vi "ComputePoint.vi"(7 "Calibration":T2={"XHP ChirpGain"=1.0, "YHP ChirpGain"=1.0, "XLP ChirpGain"=1.0, "YLP ChirpGain"=1.0}, 8 "LP Center Frequency":u32=805306367 format="%x", 9 "HP Center Frequency":u32=805306367 format="%x", 10 "UpdatesPerPoint":u32, 11 "Point":cluster{"X":i32, "Y":i32, "Z":i32} {"Y" format="%x"; "X" format="%x"}) -> (3 "settings":T1)   [LabVIEW 2011]
uses:
  AODCalibration.ctl
  CoordinateSettings.ctl
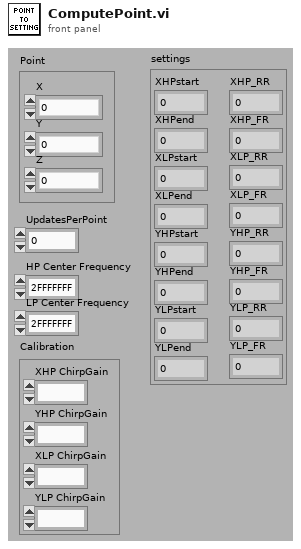
[diagram p1: front panel]
types:
  T1 = typedef "CoordinateSettings.ctl" = cluster{"XHPstart":u32, "XHPend":u32, "XLPstart":u32, "XLPend":u32, "YHPstart":u32, "YHPend":u32, "YLPstart":u32, "YLPend":u32, "XHP_RR":u32, "XHP_FR":u32, "XLP_FR":u32, "XLP_RR":u32, "YHP_FR":u32, "YHP_RR":u32, "YLP_FR":u32, "YLP_RR":u32}
  T2 = typedef "AODCalibration.ctl" = cluster{"XHP ChirpGain":fxp<+/-,16,2>, "YHP ChirpGain":fxp<+/-,16,2>, "XLP ChirpGain":fxp<+/-,16,2>, "YLP ChirpGain":fxp<+/-,16,2>}
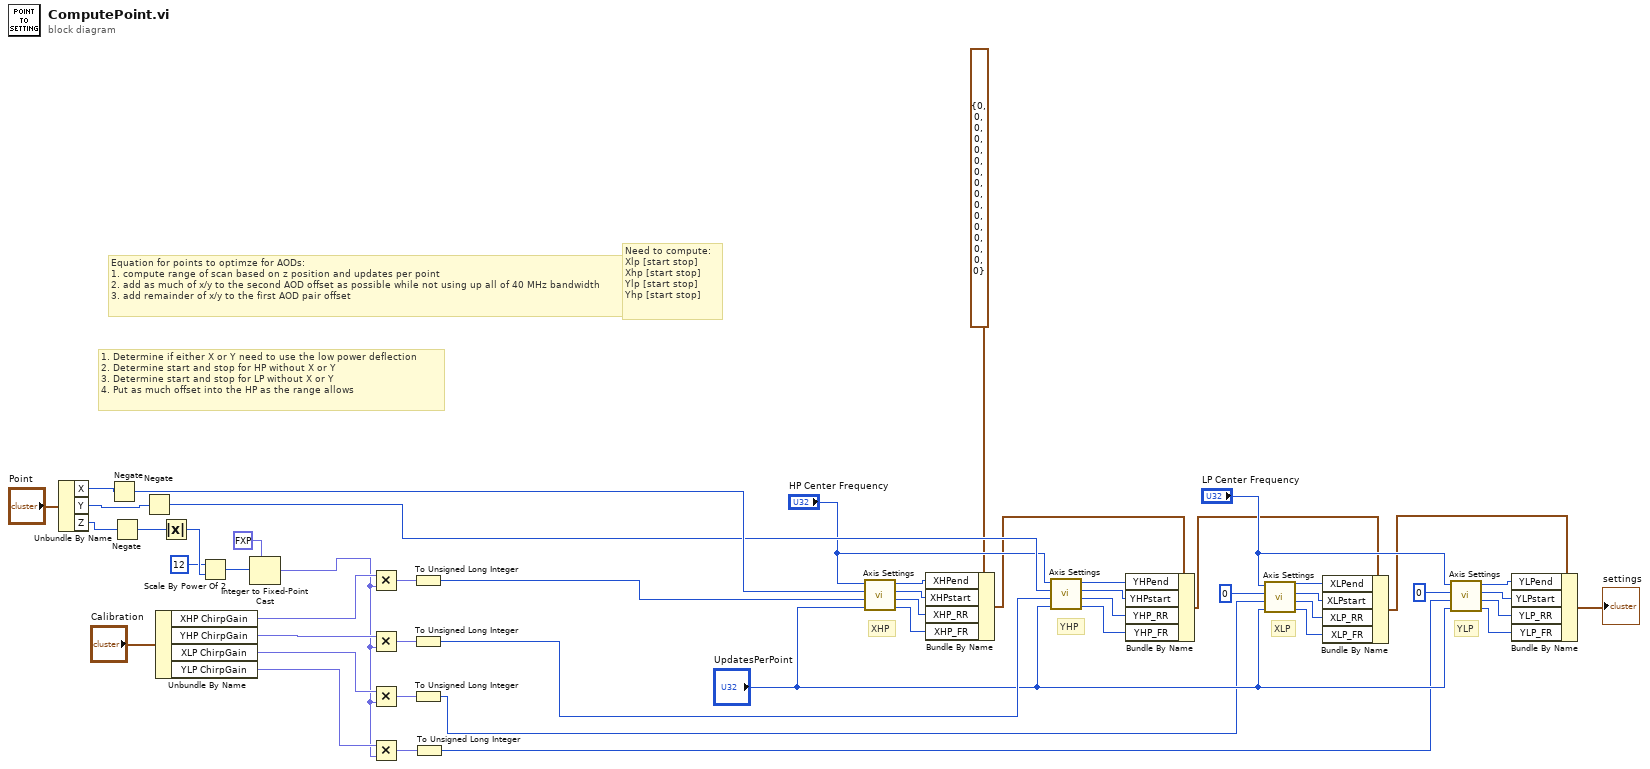
[diagram p0: block diagram]
diagram:
  # "YLP"
  # "XLP"
  # "YHP"
  # "XHP"
  # "1. Determine if either X or Y need to use the low power deflection\n2. Determine start and stop for HP without X or Y\n3. Determine start and stop for LP without X or Y\n4. Put as much offset into the HP as the range allows"
  # "Need to compute:\nXlp [start stop]\nXhp [start stop]\nYlp [start stop]\nYhp [start stop]"
  # "Equation for points to optimze for AODs:\n1. compute range of scan based on z position and updates per point\n2. add as much of x/y to the second AOD offset as possible while not using up all of 40 MHz bandwidth\n3. add remainder of x/y to the first AOD pair offset"
  n1 = Unbundle By Name("Point") -> ("X"=w50:i32, "Y"=w49:i32, "Z"=w48:i32)
  n2 = Negate(x=w50) -> (-x=w37:i32)
  n3 = Negate(x=w48) -> (-x=w42:i32)
  n4 = Negate(x=w49) -> (-x=w36:i32)
  n5 = Unbundle By Name("Calibration") -> ("XHP ChirpGain"=w46:fxp<+/-,16,2>, "YHP ChirpGain"=w45:fxp<+/-,16,2>, "XLP ChirpGain"=w44:fxp<+/-,16,2>, "YLP ChirpGain"=w43:fxp<+/-,16,2>)
  n6 = Absolute Value(x=w42) -> (abs(x)=w5:i32)
  n7 = Scale By Power Of 2(n=12, x=w5) -> (x*2^n=w3:i32)
  n8 = Integer to Fixed-Point Cast(fixed-point type=fxp<+/-,32,20> 0.0, integer=w3) -> (fixed-point=w2:fxp<+/-,32,20>)
  n9 = Multiply(x=w46, y=w2) -> (x*y=w41:fxp<+/-,48,22>)
  n10 = Multiply(x=w45, y=w2) -> (x*y=w40:fxp<+/-,48,22>)
  n11 = Multiply(x=w44, y=w2) -> (x*y=w39:fxp<+/-,48,22>)
  n12 = Multiply(x=w43, y=w2) -> (x*y=w38:fxp<+/-,48,22>)
  n13 = To Unsigned Long Integer(number=w41) -> (unsigned 32bit integer=w29:u32)
  n14 = To Unsigned Long Integer(number=w40) -> (unsigned 32bit integer=w28:u32)
  n15 = To Unsigned Long Integer(number=w39) -> (unsigned 32bit integer=w24:u32)
  n16 = To Unsigned Long Integer(number=w38) -> (unsigned 32bit integer=w22:u32)
  n17 = call "Axis Settings.vi"("Updates Per Point"="UpdatesPerPoint", "Ramp"=w29, "Offset"=w37, "Center Frequency"="HP Center Frequency") -> ("Falling Rate"=w30:u32, "Rising Rate"=w31:u32, "Low"=w32:u32, "High"=w33:u32)  [unwired: 4 in]
  n18 = Bundle By Name(cluster=T1 {"XHPstart"=0, "XHPend"=0, "XLPstart"=0, "XLPend"=0, "YHPstart"=0, "YHPend"=0, "YLPstart"=0, "YLPend"=0, "XHP_RR"=0, "XHP_FR"=0, "XLP_FR"=0, "XLP_RR"=0, "YHP_FR"=0, "YHP_RR"=0, "YLP_FR"=0, "YLP_RR"=0} ("settings"), "XHPend"=w33, "XHPstart"=w32, "XHP_RR"=w31, "XHP_FR"=w30) -> (w17:T1)
  n19 = call "Axis Settings.vi"("Updates Per Point"="UpdatesPerPoint", "Ramp"=w28, "Offset"=w36, "Center Frequency"="HP Center Frequency") -> ("Falling Rate"=w18:u32, "Rising Rate"=w19:u32, "Low"=w20:u32, "High"=w21:u32)  [unwired: 4 in]
  n20 = Bundle By Name(cluster=w17, "YHPend"=w21, "YHPstart"=w20, "YHP_RR"=w19, "YHP_FR"=w18) -> (w16:T1)
  n21 = call "Axis Settings.vi"("Updates Per Point"="UpdatesPerPoint", "Ramp"=w24, "Offset"=0, "Center Frequency"="LP Center Frequency") -> ("Falling Rate"=w12:u32, "Rising Rate"=w13:u32, "Low"=w14:u32, "High"=w15:u32)  [unwired: 4 in]
  n22 = Bundle By Name(cluster=w16, "XLPend"=w15, "XLPstart"=w14, "XLP_RR"=w13, "XLP_FR"=w12) -> (w11:T1)
  n23 = call "Axis Settings.vi"("Updates Per Point"="UpdatesPerPoint", "Ramp"=w22, "Offset"=0, "Center Frequency"="LP Center Frequency") -> ("Falling Rate"=w7:u32, "Rising Rate"=w8:u32, "Low"=w9:u32, "High"=w10:u32)  [unwired: 4 in]
  n24 = Bundle By Name(cluster=w11, "YLPend"=w10, "YLPstart"=w9, "YLP_RR"=w8, "YLP_FR"=w7) -> (→"settings":T1)
